vi "Get JSON string.vi"(8 "error in (no error)":errorcluster, 11 "File interpreter in":refnum<class "File interpreter.lvclass">) -> (0 "error out":errorcluster, 2 "String":string, 3 "File interpreter out":refnum<class "File interpreter.lvclass">)   [LabVIEW 2018, in "File interpreter.lvclass"]
uses:
  File interpreter.lvclass
  File interpreter.lvclass/File interpreter.ctl
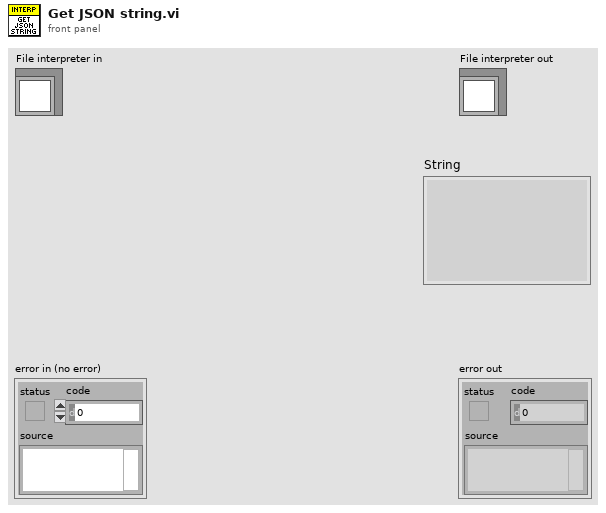
[diagram p1: front panel]
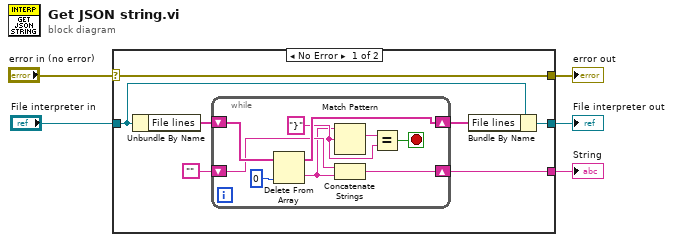
[diagram p0: block diagram]
diagram:
  n1 = case shown="No Error" "error in (no error)" {
    selector: "error in (no error)" -> [w12 w23]
    tunnel: [w12 w23] -> w4
    tunnel: [w10 w22] -> w2
    tunnel: "File interpreter in" -> [w11 w22]
    tunnel: [w8 _] -> w1
    frame No Error {
      n2 = Unbundle By Name(w11) -> ("File lines"=w6:string[])
      n3 = while {
        shift-right: [w20] -> w7
        shift-left: w6 -> [w21]
        shift-right: [w14] -> w8
        shift-left: "" -> [w15]
        stop <- w18 stop-if-true
        w16 = "}"
        n4 = Delete From Array(array=w21, index=0) -> (deleted portion=w13:string, array with subset deleted=w20:string[])  [unwired: 1 in]
        n5 = Match Pattern(string=w13, regular expression=w16) -> (match substring=w17:string)  [unwired: 1 in, 3 out]
        n6 = Concatenate Strings(w15, w13) -> (w14:string)
        n7 = Equal?(x=w17, y=w16) -> (x = y?=w18:bool)
      }
      n8 = Bundle By Name(cluster=w11, "File lines"=w7) -> (w10:refnum<class "File interpreter.lvclass">)
    }
    frame Error {
    }
  }
  "error out" <- w4
  "File interpreter out" <- w2
  "String" <- w1
